vi "scope Oct27 2017.vi"() -> ()   [LabVIEW 2014]
uses:
  <instrlib>/Tektronix TDS 200 1000 2000 Series/Public/Data/Read (Single Waveform).vi
  <vilib>/Utility/file.llb/Write To Spreadsheet File (string).vi
  <instrlib>/Tektronix TDS 200 1000 2000 Series/Tektronix TDS 200 1000 2000 Series.lvlib
panel:
  out "output":string[][](array[string])
  in  "milliseconds to wait":u32=10000
  out "File path 2":path
  in  "sweep number":i32
  in  "begin sweep":bool
  out "Waveform Graph 2":waveform(dbl)(graph)
  out "Waveform Graph":waveform(dbl)(graph)
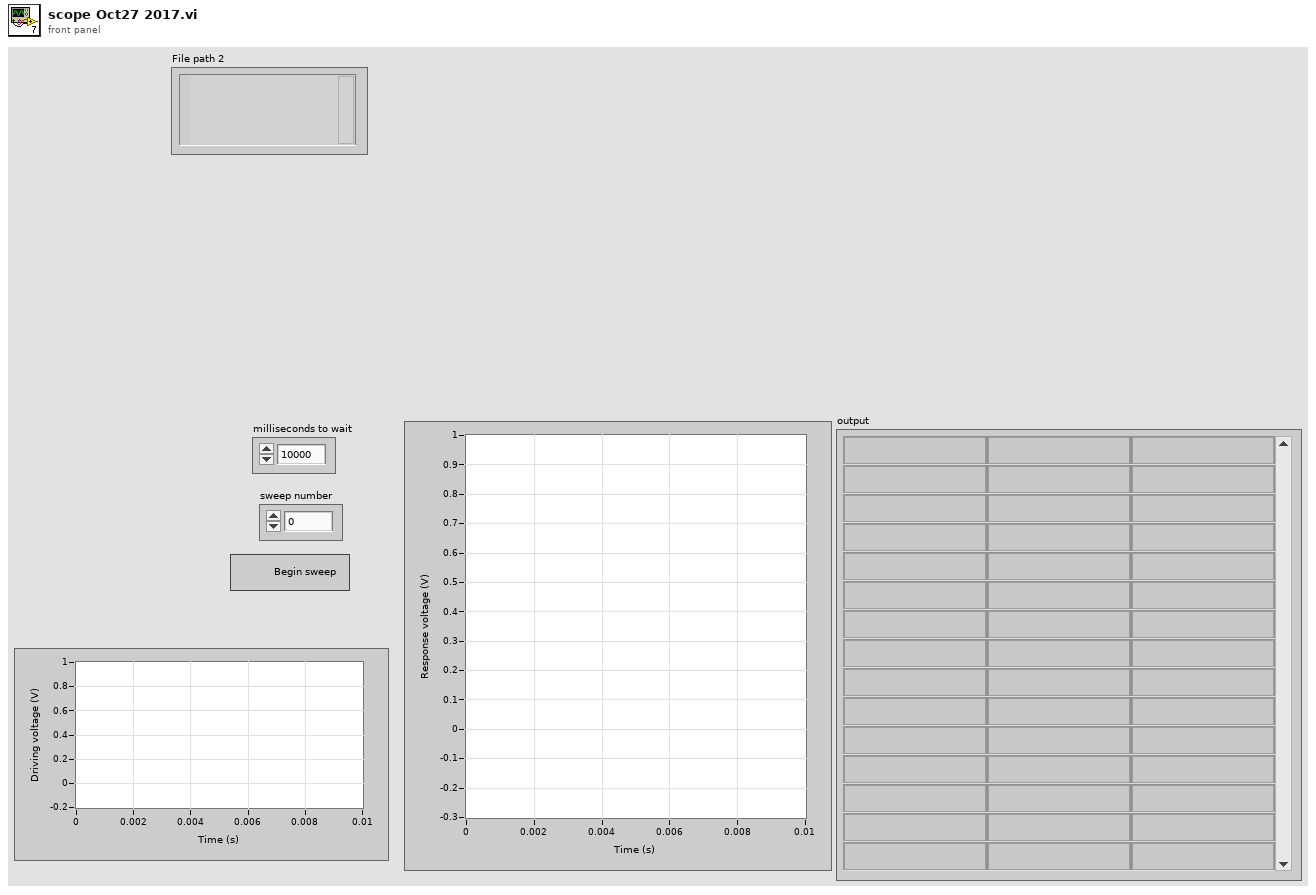
[diagram p1: front panel]
types:
  T1 = enum16{"open", "open or create", "create or replace", "create", "open (read only)"}
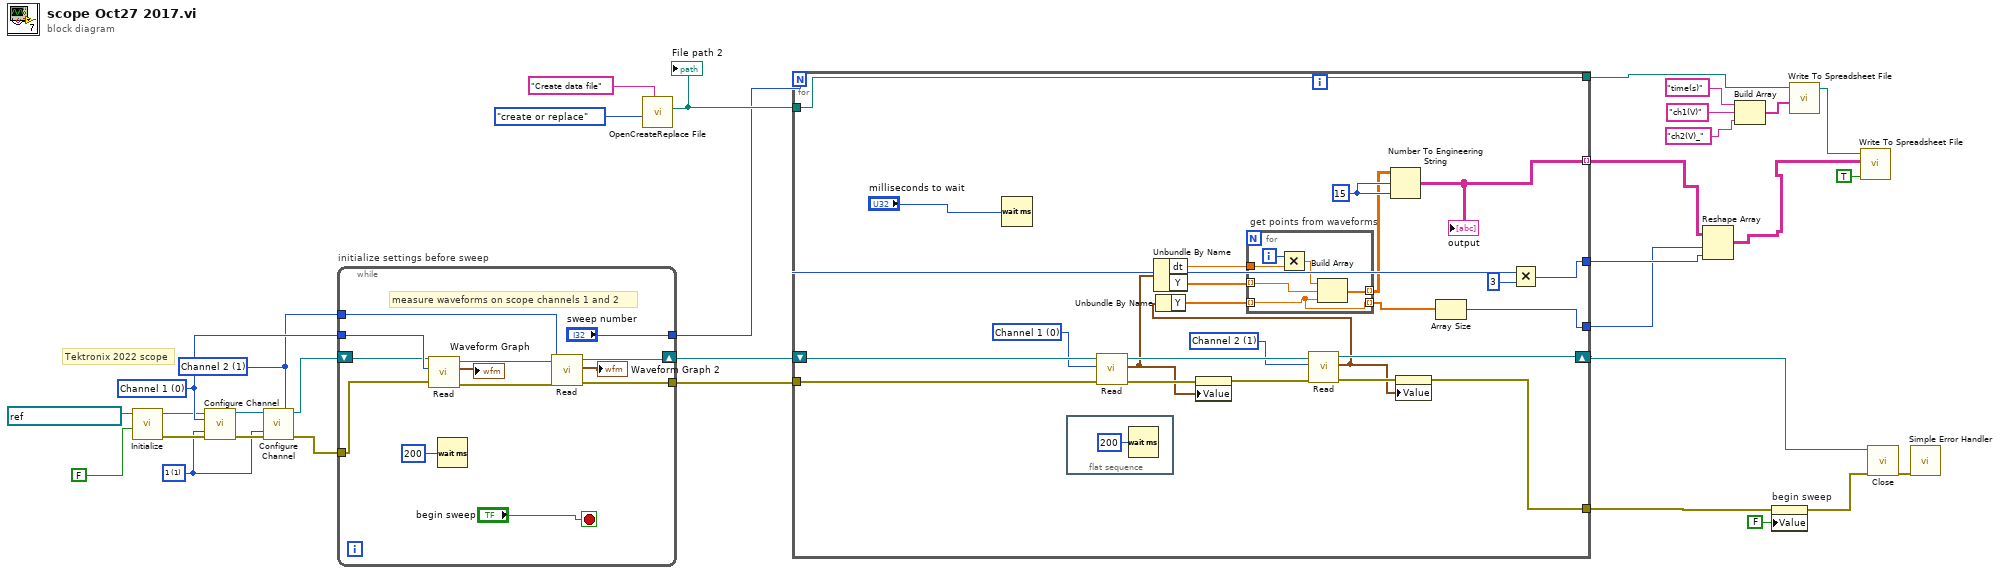
[diagram p0: block diagram]
diagram:
  w21 = 1 items=["1"=1, "10"=10, "20"=20, "50"=50, "100"=100, "500"=500, "1000"=1000] ("Probe Attenuation (10: 10X)")
  w24 = 0 items=["Channel 1", "Channel 2", "Channel 3", "Channel 4", "Math", "Reference A", "Reference B", "Reference C", "Reference D"] ("Channel (0: Channel 1)")
  w23 = 1 items=["Channel 1", "Channel 2", "Channel 3", "Channel 4", "Math", "Reference A", "Reference B", "Reference C", "Reference D"] ("Channel (0: Channel 1)")
  # "Tektronix 2022 scope"
  n1 = call <instrlib>:"Initialize.vi"("Reset? (T: Yes)"=FALSE, "VISA resource name"=refnum<visa-resource-name> "GPIB1::20::INSTR") -> ("error out"=w27:errorcluster, "VISA resource name out"=w22:refnum<visa-resource-name>)  [unwired: 8 in]
  n2 = call <instrlib>:"Configure Channel.vi"("VISA resource name"=w22, "Channel (0: Channel 1)"=w24, "Probe Attenuation (10: 10X)"=w21, "error in (no error)"=w27) -> ("VISA resource name out"=w28:refnum<visa-resource-name>, "error out"=w26:errorcluster)  [unwired: 10 in]
  n3 = call <instrlib>:"Configure Channel.vi"("VISA resource name"=w28, "Channel (0: Channel 1)"=w23, "Probe Attenuation (10: 10X)"=w21, "error in (no error)"=w26) -> ("VISA resource name out"=w25:refnum<visa-resource-name>, "error out"=w18:errorcluster)  [unwired: 10 in]
  n4 = while "initialize settings before sweep" {
    shift-right: [w40] -> w31
    shift-left: w25 -> [w41]
    tunnel: w24 -> [w45]
    tunnel: w23 -> [w44]
    tunnel: w18 -> [w37]
    tunnel: [w36] -> w16
    tunnel: ["sweep number"] -> w11
    stop <- "begin sweep" stop-if-true
    # "measure waveforms on scope channels 1 and 2"
    n5 = call-poly <instrlib>:"Read.vi"("error in (no error)"=w37, "Source (0: Channel 1)"=w45, "VISA resource name"=w41) -> ("error out"=w42:errorcluster, "Waveform Data"=→"Waveform Graph":waveform(dbl), "VISA resource name out"=w43:refnum<visa-resource-name>)  [unwired: 6 in]
    n6 = Wait (ms)(milliseconds to wait=u32 200) -> ()  [unwired: 1 out]
    n7 = call-poly <instrlib>:"Read.vi"("error in (no error)"=w42, "Source (0: Channel 1)"=w44, "VISA resource name"=w43) -> ("error out"=w36:errorcluster, "Waveform Data"=→"Waveform Graph 2":waveform(dbl), "VISA resource name out"=w40:refnum<visa-resource-name>)  [unwired: 6 in]
  }
  n8 = call "OpenCreateReplace File.vi"("prompt"="Create data file", "function (open:0)"=T1."create or replace") -> ("new file path"=w13:path)  [unwired: 6 in, 3 out]
  "File path 2" <- w13
  n9 = for "Number of sweeps per amplitude" {
    N: w11 -> [w52]
    tunnel: [w70] -> w32
    tunnel: w16 -> [w71]
    shift-right: [w68] -> w30
    shift-left: w31 -> [w69]
    tunnel: w13 -> [w54]
    tunnel: [w53] -> w10 mode=indexing
    tunnel: [w54] -> w6
    tunnel: [w50] -> w8
    tunnel: [w47] -> w7
    w58 = i16 15 ("precision (6)")
    w64 = 1 items=["Channel 1", "Channel 2", "Channel 3", "Channel 4", "Math", "Reference A", "Reference B", "Reference C", "Reference D"] ("Channel (0: Channel 1)")
    w65 = 0 items=["Channel 1", "Channel 2", "Channel 3", "Channel 4", "Math", "Reference A", "Reference B", "Reference C", "Reference D"] ("Channel (0: Channel 1)")
    n10 = Wait (ms)(milliseconds to wait="milliseconds to wait") -> ()  [unwired: 1 out]
    n11 = flat-sequence {
      frame #0 {
        n12 = Wait (ms)(milliseconds to wait=u32 200) -> ()  [unwired: 1 out]
      }
    }
    n13 = call-poly <instrlib>:"Read.vi"("error in (no error)"=w71, "Source (0: Channel 1)"=w65, "VISA resource name"=w69) -> ("error out"=w63:errorcluster, "Waveform Data"=w56:waveform(dbl), "VISA resource name out"=w66:refnum<visa-resource-name>)  [unwired: 6 in]
    n14 = Unbundle By Name(w56) -> ("dt"=w60:dbl, "Y"=w57:dbl[])
    n15 = property on="Waveform Graph" class="WFGraph (strict)"(error in=w63, "Value"=w56) -> (error out=w62:errorcluster)  [unwired: 1 in, 1 out]
    n16 = call-poly <instrlib>:"Read.vi"("error in (no error)"=w62, "Source (0: Channel 1)"=w64, "VISA resource name"=w66) -> ("error out"=w61:errorcluster, "Waveform Data"=w55:waveform(dbl), "VISA resource name out"=w68:refnum<visa-resource-name>)  [unwired: 6 in]
    n17 = Unbundle By Name(w55) -> ("Y"=w59:dbl[])
    n18 = for "get points from waveforms" {
      tunnel: w60 -> [w76]
      tunnel: w57 -> [w74] mode=indexing
      tunnel: [w73] -> w49 mode=indexing
      tunnel: w59 -> [w72] mode=indexing
      tunnel: [w72] -> w48 mode=indexing
      i -> [w77]
      n19 = Multiply(x=w77, y=w76) -> (x*y=w75:dbl)
      n20 = Build Array(w75, w74, w72) -> (w73:dbl[])
    }
    n21 = Number To Engineering String(2:w58, 3:w58, 4:w49) -> (0:w53:string[][])  [unwired: 1 in]
    "output" <- w53
    n22 = property on="Waveform Graph 2" class="WFGraph (strict)"(error in=w61, "Value"=w55) -> (error out=w70:errorcluster)  [unwired: 1 in, 1 out]
    n23 = Array Size(array=w48) -> (size(s)=w47:i32)
    n24 = Multiply(x=w52, y=3) -> (x*y=w50:i32)
  }
  n25 = Reshape Array(w10, w7, w8) -> (w9:string[][])
  n26 = Build Array("time(s)", "ch1(V)", "ch2(V)_") -> (w1:string[])
  n27 = property on="begin sweep" class="Bool (strict)"(error in=w32, "Value"=FALSE ("begin sweep")) -> (error out=w20:errorcluster)  [unwired: 1 in, 1 out]
  n28 = call-poly <vilib>:"Write To Spreadsheet File.vi"("1D data"=w1, "file path (dialog if empty)"=w6) -> ("new file path (Not A Path if cancelled)"=w5:path)  [unwired: 6 in]
  n29 = call-poly <vilib>:"Write To Spreadsheet File.vi"("append to file? (new file:F)"=TRUE, "2D data"=w9, "file path (dialog if empty)"=w5) -> ()  [unwired: 5 in, 1 out]
  n30 = call <instrlib>:"Close.vi"("error in (no error)"=w20, "VISA resource name"=w30) -> ("error out"=w19:errorcluster)  [unwired: 9 in]
  n31 = call <vilib>:"Simple Error Handler.vi"("error in (no error)"=w19) -> ()  [unwired: 4 in, 5 out]
